vi "ACT L_bank_Control_06.vi"(0 "SI804.lvclass in":refnum<class "SI804.lvclass">, 1 "3 JSA20 DT104\nXA01":bool, 2 "3 JSA20 DT105\nXA01":bool, 5 "error in":errorcluster) -> (14 "SI804.lvclass out":refnum<class "SI804.lvclass">, 16 "ACT-Ctrl\nL-bank 1/2 insertion":bool, 17 "ACT-Ctrl\nL-bank 1/2 withdrawal":bool, 19 "error out":errorcluster)   [LabVIEW 2022 SP3, in "SI804.lvclass"]
uses:
  SI804.lvclass
  SI804.lvclass/SI804.ctl
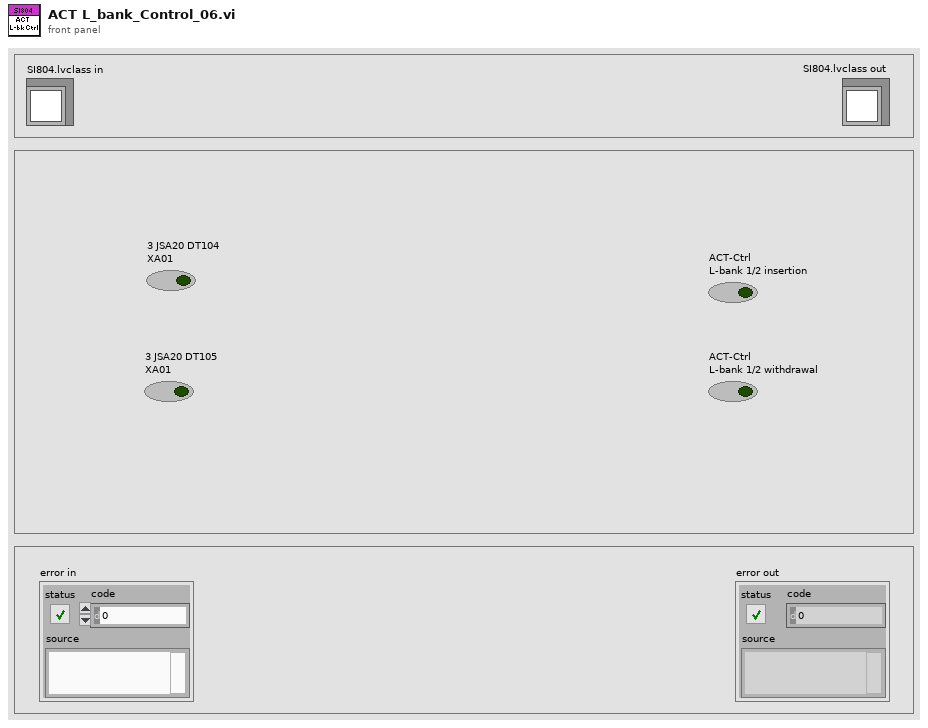
[diagram p1: front panel]
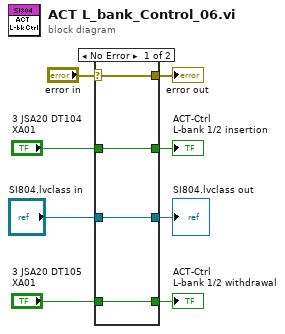
[diagram p0: block diagram]
diagram:
  n1 = case shown="No Error" "error in" {
    selector: "error in" -> [w9 w14]
    tunnel: "3 JSA20 DT104\nXA01" -> [w11 _]
    tunnel: "3 JSA20 DT105\nXA01" -> [w10 _]
    tunnel: "SI804.lvclass in" -> [w12 w13]
    tunnel: [w12 w13] -> w4
    tunnel: [w11 _] -> w2
    tunnel: [w10 _] -> w1
    tunnel: [w9 w14] -> w3
    frame No Error {
    }
    frame Error {
    }
  }
  "SI804.lvclass out" <- w4
  "error out" <- w3
  "ACT-Ctrl\nL-bank 1/2 insertion" <- w2
  "ACT-Ctrl\nL-bank 1/2 withdrawal" <- w1
